vi "Translator.FindVi.vi"(8 "error in":errorcluster, 10 "VI name":string) -> (0 "error out":errorcluster, 1 "find":bool, 2 "Array":string[](array[string]))   [LabVIEW 2014]
panel:
  out "Application:All VIs In Memory":string[](array[string])
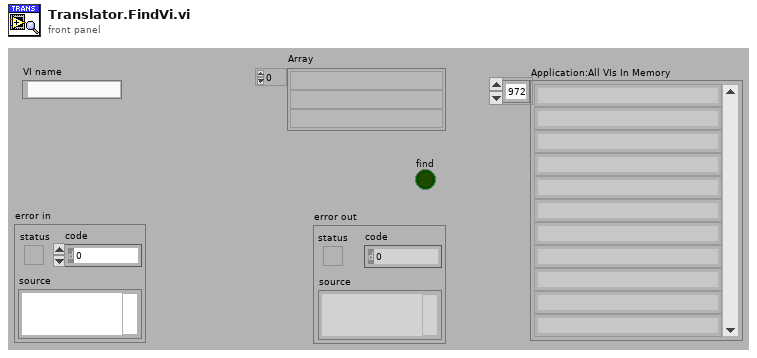
[diagram p1: front panel]
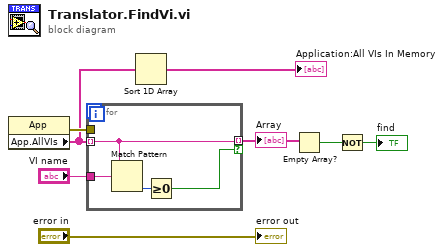
[diagram p0: block diagram]
diagram:
  n1 = property class="App"() -> (error out=w7:errorcluster, "App.AllVIs"=w2:string[])  [unwired: 2 in, 1 out]
  n2 = for {
    tunnel: w2 -> [w10] mode=indexing
    tunnel: "VI name" -> [w12]
    tunnel: w7 -> [_]
    tunnel: [w10] -> w5 mode=indexing if=w9
    n3 = Match Pattern(string=w10, regular expression=w12) -> (offset past match=w11:i32)  [unwired: 1 in, 3 out]
    n4 = Greater Or Equal To 0?(x=w11) -> (x >= 0?=w9:bool)
  }
  "Array" <- w5
  n5 = Sort 1D Array(array=w2) -> (sorted array=→"Application:All VIs In Memory":string[])
  n6 = Empty Array?(array=w5) -> (empty?=w4:bool)
  n7 = Not(x=w4) -> (.not. x?=→"find":bool)
  "error out" <- "error in"
